vi "FlatToRichnixnet_grpc_DbCreateObjectResponse.vi"(5 "OutputClusterType":T1, 11 "InputCluster":T3) -> (3 "OutputCluster":T1)   [LabVIEW 2025, in "xnet-grpc_client.lvlib"]
uses:
  xnet-grpc_client.lvlib
  nixnet_grpc_DbCreateObjectResponse_Flat.ctl
  nidevice_grpc_Session_Flat.ctl
  nixnet_grpc_DbCreateObjectResponse.ctl
  nidevice_grpc_Session.ctl
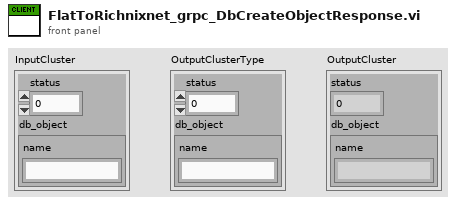
[diagram p1: front panel]
types:
  T1 = typedef "xnet-grpc_client.lvlib/nixnet_grpc_DbCreateObjectResponse.ctl" = cluster{"status":i32, "db_object":T2}
  T2 = typedef "xnet-grpc_client.lvlib/nidevice_grpc_Session.ctl" = cluster{"name":string}
  T3 = typedef "xnet-grpc_client.lvlib/nixnet_grpc_DbCreateObjectResponse_Flat.ctl" = cluster{"status":i32, "db_object":T4}
  T4 = typedef "xnet-grpc_client.lvlib/nidevice_grpc_Session_Flat.ctl" = cluster{"name":string}
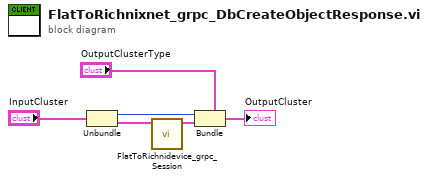
[diagram p0: block diagram]
diagram:
  n1 = Unbundle "Unbundle"("InputCluster") -> ("status"=w3:i32, "db_object"=w2:T4)
  n2 = call "FlatToRichnidevice_grpc_Session.vi"("InputCluster"=w2) -> ("OutputCluster"=w1:T2)  [unwired: 10 in]
  n3 = Bundle "Bundle"(cluster="OutputClusterType", "status"=w3, "db_object"=w1) -> (→"OutputCluster":T1)
